vi "Get Integrated Area.vi"(8 "error in":errorcluster, 10 "p":i32=1, 11 "PAS Cell Data in":refnum<class "PAS Cell Data.lvclass">) -> (0 "error out":errorcluster, 3 "PAS Cell Data out":refnum<class "PAS Cell Data.lvclass">)   [LabVIEW 2015, in "PAS Cell Data.lvclass"]
doc: "This VI takes an input frequency signal and 1) sets a noise threshold (the value below which the spectrum resembles white noise) , 2) sets bounds over which to integrate, 3) finds the integrated area and 4) returns that integrated area with the noise below the threshold level defined by <B>P</B> removed."
uses:
  PAS Cell Data.lvclass
  PAS Cell Data.lvclass/PAS Cell Data.ctl
  General/Math Utilities.lvlib
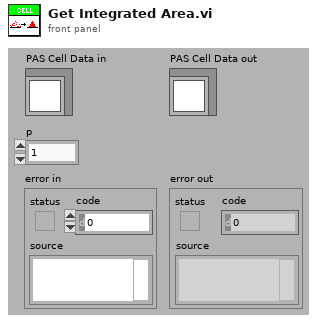
[diagram p1: front panel]
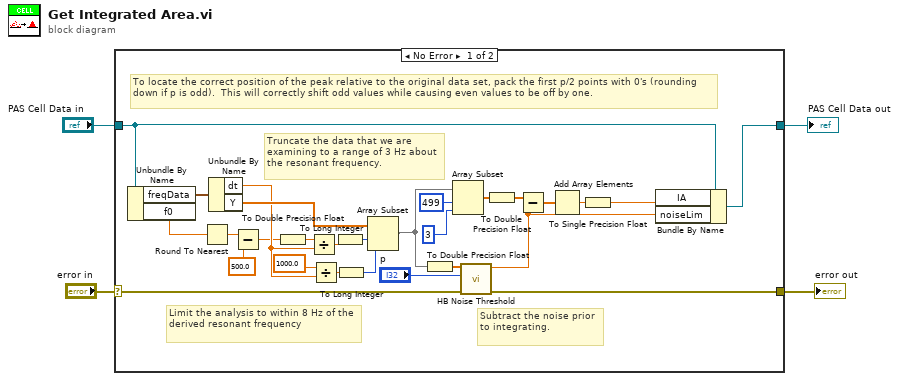
[diagram p0: block diagram]
diagram:
  n1 = case shown="No Error" "error in" {
    selector: "error in" -> [w24 w34]
    tunnel: [w20 w34] -> w3
    tunnel: [w22 w33] -> w1
    tunnel: "PAS Cell Data in" -> [w7 w33]
    frame No Error {
      # "Truncate the data that we are examining to a range of 3 Hz about the resonant frequency."
      # "To locate the correct position of the peak relative to the original data set, pack the first p/2 points with 0's (rounding down if p is odd).  This will correctly shift odd values while causing even values to be off by one."
      # "Subtract the noise prior to integrating."
      # "Limit the analysis to within 8 Hz of the derived resonant frequency"
      n2 = Unbundle By Name(w7) -> ("freqData"=w26:waveform(sgl), "f0"=w25:sgl)
      n3 = Round To Nearest(number=w25) -> (nearest integer value=w30:sgl)
      n4 = Unbundle By Name(w26) -> ("dt"=w23:dbl, "Y"=w29:sgl[])
      n5 = Subtract(x=w30, y=sgl 500.0) -> (x-y=w13:sgl)
      n6 = To Double Precision Float(number=w13) -> (double precision float=w14:dbl)
      n7 = Divide(x=w14, y=w23) -> (x/y=w17:dbl)
      n8 = Divide(x=1000.0, y=w23) -> (x/y=w15:dbl)
      n9 = To Long Integer(number=w17) -> (32bit integer=w18:i32)
      n10 = To Long Integer(number=w15) -> (32bit integer=w16:i32)
      n11 = Array Subset(array=w29, index=w18, length=w16) -> (w11:sgl[])
      n12 = To Double Precision Float(number=w11) -> (double precision float=w10:dbl[])
      n13 = Array Subset(array=w11, index=499, length=3) -> (w8:sgl[])
      n14 = call "HB Noise Threshold.vi"("Error In"=w24, "p"="p", "Y"=w10) -> ("Error Out"=w20:errorcluster, "P"=w19:dbl)  [unwired: 7 out]
      n15 = To Double Precision Float(number=w8) -> (double precision float=w9:dbl[])
      n16 = Subtract(x=w9, y=w19) -> (x-y=w31:dbl[])
      n17 = Add Array Elements(numeric array=w31) -> (sum=w6:dbl)
      n18 = To Single Precision Float(number=w6) -> (single precision float=w5:sgl)
      n19 = Bundle By Name(cluster=w7, "IA"=w5, "noiseLim"=w19) -> (w22:refnum<class "PAS Cell Data.lvclass">)
    }
    frame Error {
    }
  }
  "error out" <- w3
  "PAS Cell Data out" <- w1
